vi "Magnetometer_Test_ReportGenerator.vi"() -> ()   [LabVIEW 2019]
uses:
  <vilib>/Utility/file.llb/Write Delimited Spreadsheet (string).vi
panel:
  in  "stop":bool
  out "error out":errorcluster
  out "Time 2":string
  out "X-Axis 2":string
  out "Time":string
  out "X-Axis":string
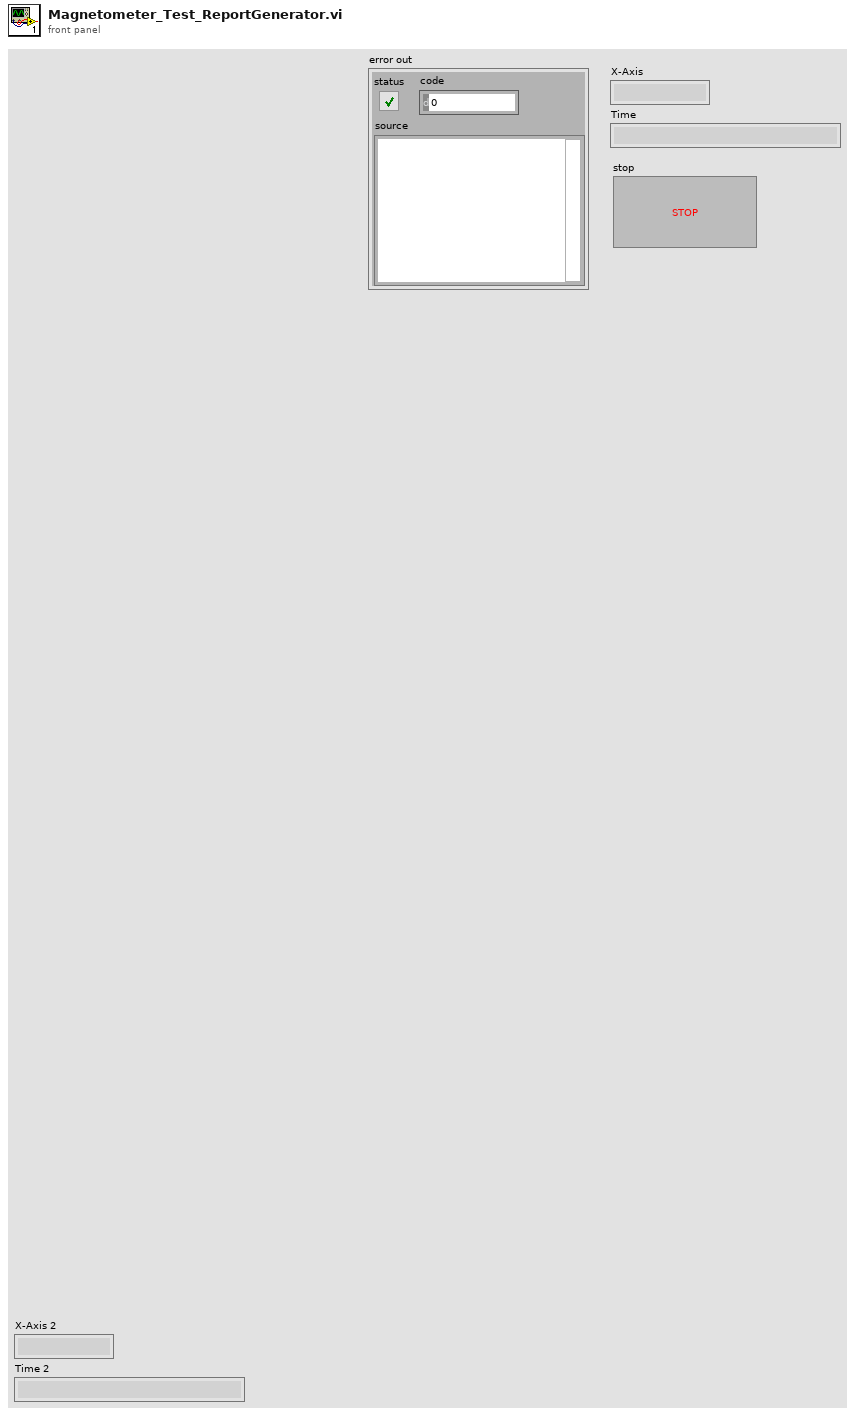
[diagram p1: front panel]
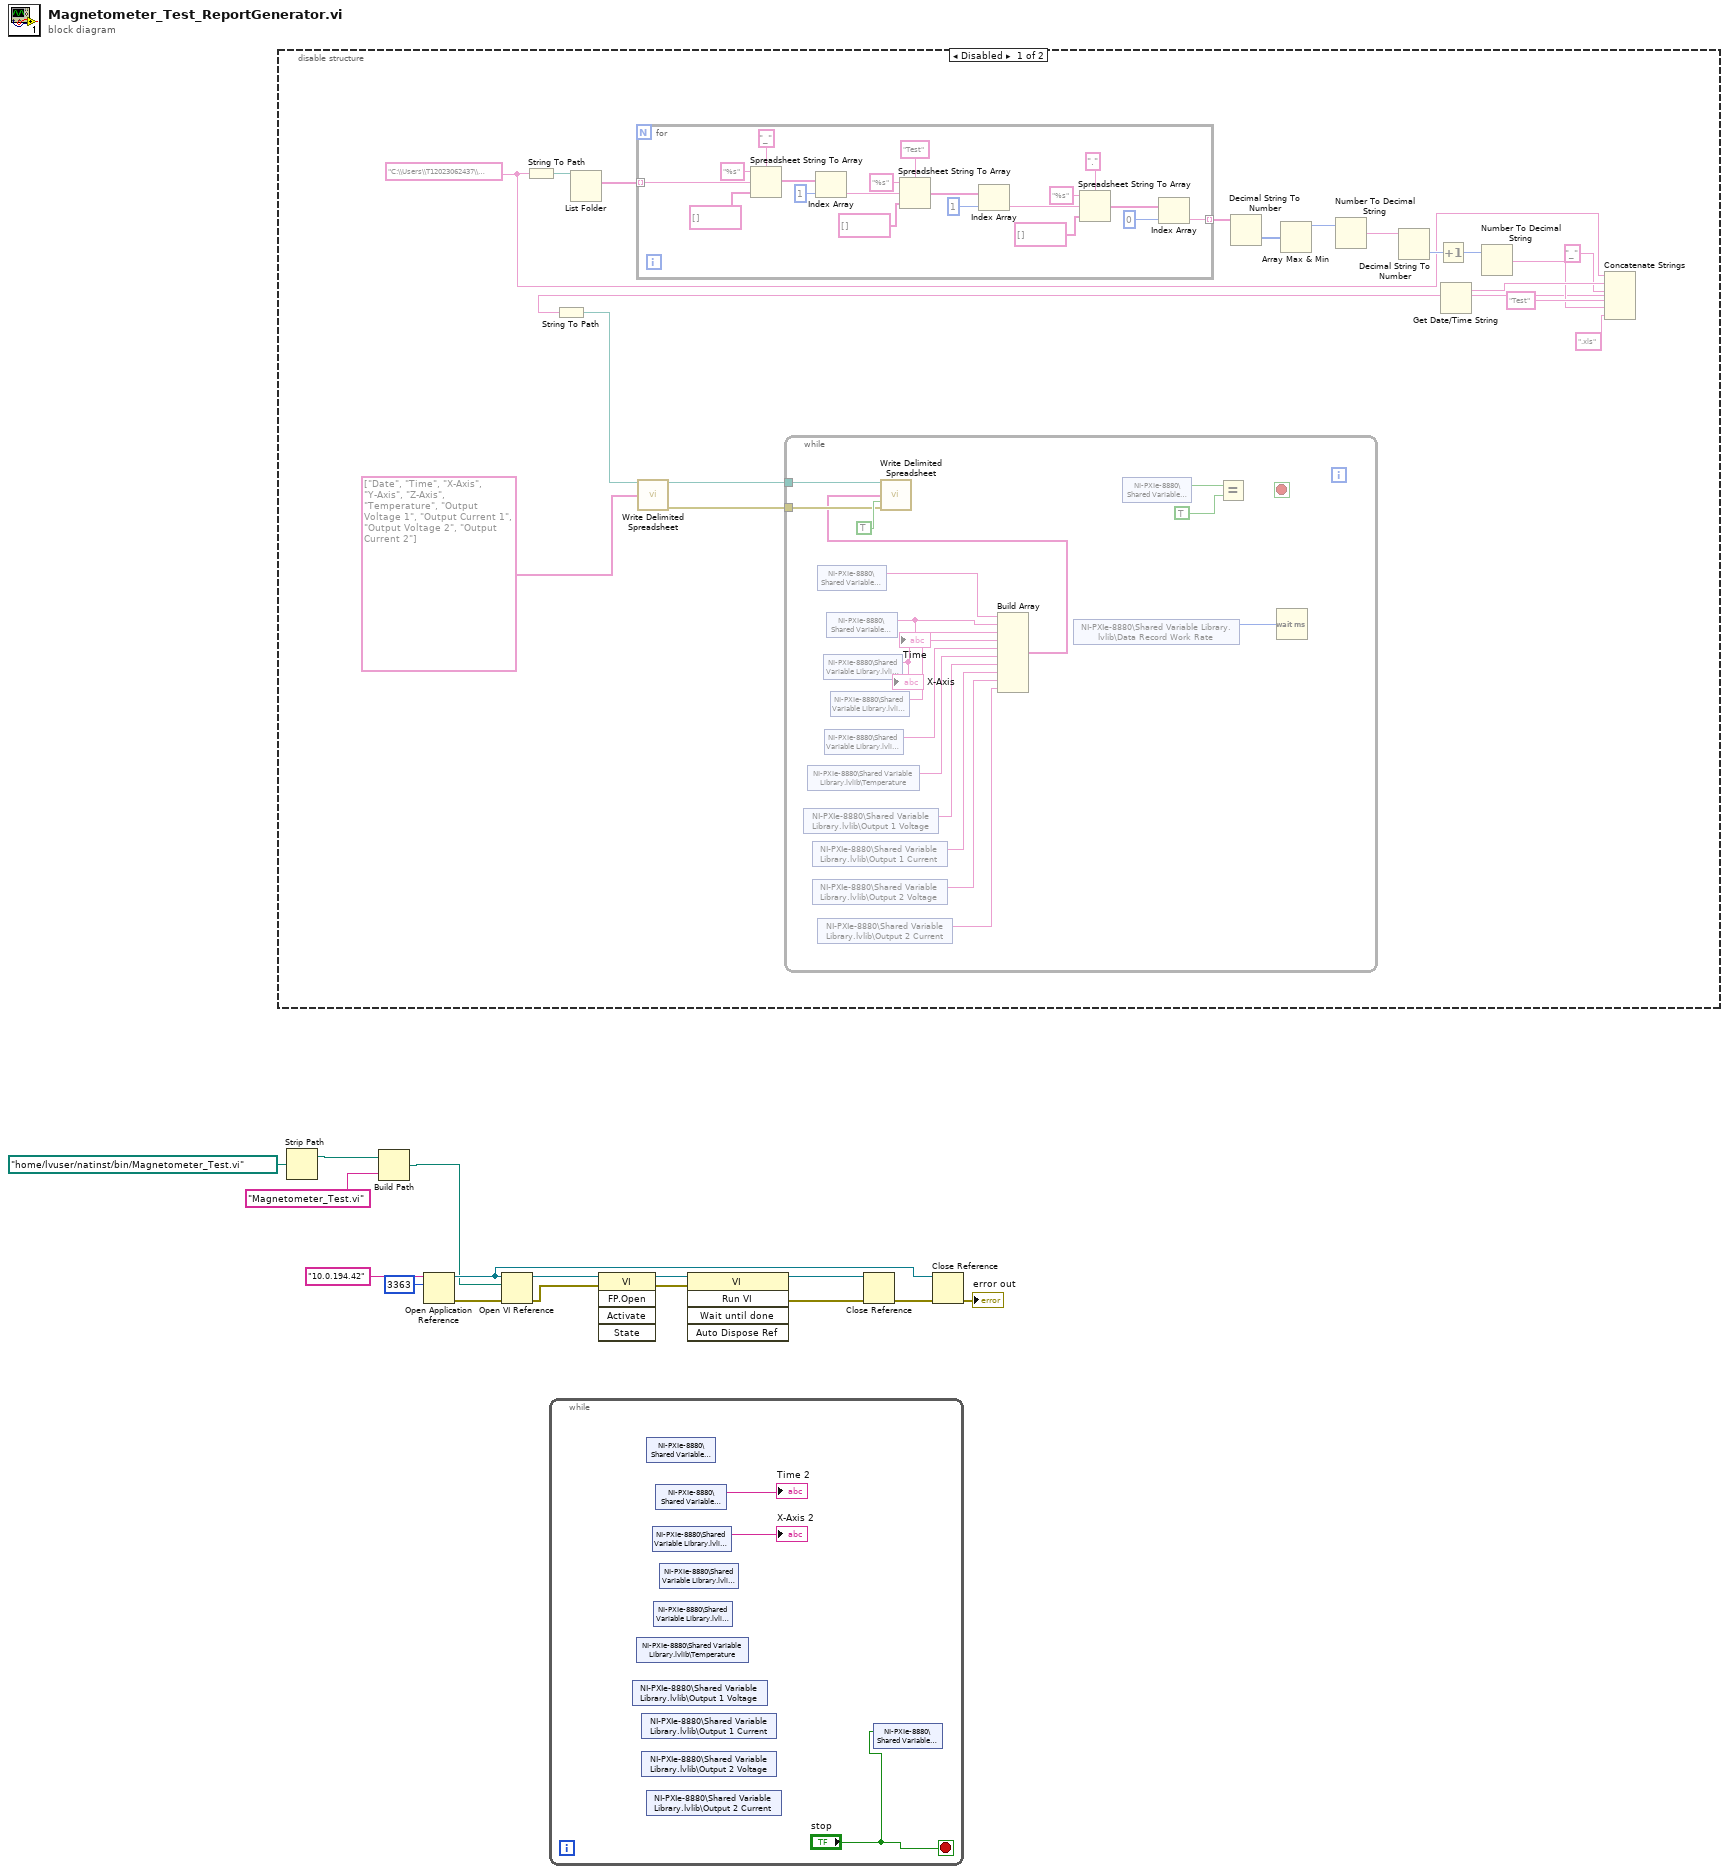
[diagram p0: block diagram]
diagram:
  n1 = disable-structure shown="Disabled" {
    frame Disabled {
      w19 = "C:\\Users\\T12023062437\\Desktop\\GKY Labview Models\\GKY Magnetometer Test Model Workspace\\Test Report\\"
      n2 = String To Path(string=w19) -> (path=w21:path)
      n3 = List Folder(path=w21) -> (filenames=w25:string[])  [unwired: 3 in, 3 out]
      n4 = for {
        tunnel: w25 -> [w39] mode=indexing
        tunnel: [w38] -> w24 mode=indexing
        n5 = Spreadsheet String To Array(delimiter (Tab)="_", format string="%s", spreadsheet string=w39, array type (2D Dbl)=string[] []) -> (array=w51:string[])
        n6 = Index Array(array=w51, index=1) -> (element=w52:string)
        n7 = Spreadsheet String To Array(delimiter (Tab)="Test", format string="%s", spreadsheet string=w52, array type (2D Dbl)=string[] []) -> (array=w36:string[])
        n8 = Index Array(array=w36, index=1) -> (element=w54:string)
        n9 = Spreadsheet String To Array(delimiter (Tab)=".", format string="%s", spreadsheet string=w54, array type (2D Dbl)=string[] []) -> (array=w53:string[])
        n10 = Index Array(array=w53, index=0) -> (element=w38:string)
      }
      n11 = Decimal String To Number(string=w24) -> (number=w23:i32[])  [unwired: 2 in, 1 out]
      n12 = Array Max & Min(array=w23) -> (max value=w22:i32)  [unwired: 3 out]
      n13 = Number To Decimal String(number=w22) -> (decimal integer string=w20:string)  [unwired: 1 in]
      n14 = Decimal String To Number(string=w20) -> (number=w30:i32)  [unwired: 2 in, 1 out]
      n15 = Increment(x=w30) -> (x+1=w29:i32)
      n16 = Get Date/Time String() -> (date string=w33:string)  [unwired: 3 in, 1 out]
      n17 = Number To Decimal String(number=w29) -> (decimal integer string=w28:string)  [unwired: 1 in]
      n18 = Concatenate Strings(w19, w33, "_" ("string"), "Test" ("string"), w28, ".xls" ("string")) -> (w27:string)
      n19 = String To Path(string=w27) -> (path=w17:path)
      n20 = call-poly <vilib>:"Write Delimited Spreadsheet.vi"("file path (dialog if empty)"=w17, "1D data"=string[] ["Date", "Time", "X-Axis", "Y-Axis", "Z-Axis", "Temperature", "Output Voltage 1", "Output Current 1", "Output Voltage 2", "Output Current 2"]) -> ("new file path (Not A Path if cancelled)"=w35:path, "error out"=w34:errorcluster)  [unwired: 12 in]
      n21 = while {
        tunnel: w35 -> [w73]
        tunnel: w34 -> [w71]
        stop <- w55 stop-if-true
        n22 = shared-variable "NI-PXIe-8880\\Shared Variable Library.lvlib\\Output 1 Voltage"() -> (w62:string)  [unwired: 1 in, 1 out]
        n23 = shared-variable "NI-PXIe-8880\\Shared Variable Library.lvlib\\Temperature"() -> (w63:string)  [unwired: 1 in, 1 out]
        n24 = shared-variable "NI-PXIe-8880\\Shared Variable Library.lvlib\\Output 1 Current"() -> (w61:string)  [unwired: 1 in, 1 out]
        n25 = shared-variable "NI-PXIe-8880\\Shared Variable Library.lvlib\\Output 2 Voltage"() -> (w60:string)  [unwired: 1 in, 1 out]
        n26 = shared-variable "NI-PXIe-8880\\Shared Variable Library.lvlib\\Date"() -> (w68:string)  [unwired: 1 in, 1 out]
        n27 = shared-variable "NI-PXIe-8880\\Shared Variable Library.lvlib\\Output 2 Current"() -> (w59:string)  [unwired: 1 in, 1 out]
        n28 = shared-variable "NI-PXIe-8880\\Shared Variable Library.lvlib\\X-Axis"() -> (w66:string)  [unwired: 1 in, 1 out]
        "X-Axis" <- w66
        n29 = shared-variable "NI-PXIe-8880\\Shared Variable Library.lvlib\\Z-Axis"() -> (w64:string)  [unwired: 1 in, 1 out]
        n30 = shared-variable "NI-PXIe-8880\\Shared Variable Library.lvlib\\Time"() -> (w67:string)  [unwired: 1 in, 1 out]
        "Time" <- w67
        n31 = shared-variable "NI-PXIe-8880\\Shared Variable Library.lvlib\\Y-Axis"() -> (w65:string)  [unwired: 1 in, 1 out]
        n32 = Build Array(w68, w67, w66, w65, w64, w63, w62, w61, w60, w59) -> (w58:string[])
        n33 = call-poly <vilib>:"Write Delimited Spreadsheet.vi"("file path (dialog if empty)"=w73, "1D data"=w58, "append to file? (new file:F)"=TRUE, "error in (no error)"=w71) -> ()  [unwired: 10 in, 2 out]
        n34 = shared-variable "NI-PXIe-8880\\Shared Variable Library.lvlib\\Data Record Work Rate"() -> (w57:u16)  [unwired: 1 in, 1 out]
        n35 = shared-variable "NI-PXIe-8880\\Shared Variable Library.lvlib\\Stop"() -> (w70:bool)  [unwired: 1 in, 1 out]
        n36 = Equal?(x=w70, y=TRUE) -> (x = y?=w56:bool)
        n37 = Wait (ms)(milliseconds to wait=w57) -> ()  [unwired: 1 out]
      }
    }
    frame Enabled {
    }
  }
  n38 = Strip Path(path=path "/home/lvuser/natinst/bin/Magnetometer_Test.vi") -> (stripped path=w5:path)  [unwired: 1 out]
  n39 = Build Path(base path=w5, name or relative path="Magnetometer_Test.vi") -> (appended path=w2:path)
  n40 = Open Application Reference(10:u16 3363 ("port number or service name (3363)"), 11:"10.0.194.42" ("machine name (\"\":  open local reference)")) -> (0:w13:errorcluster, 3:w7:refnum<vi>)  [unwired: 2 in]
  n41 = Open VI Reference(application reference (local)=w7, vi path=w2, error in (no error)=w13) -> (vi reference=w16:refnum<vi>, error out=w12:errorcluster)  [unwired: 3 in]
  n42 = while {
    stop <- "stop" stop-if-true
    n43 = shared-variable "NI-PXIe-8880\\Shared Variable Library.lvlib\\Output 1 Voltage"() -> ()  [unwired: 1 in, 2 out]
    n44 = shared-variable "NI-PXIe-8880\\Shared Variable Library.lvlib\\Temperature"() -> ()  [unwired: 1 in, 2 out]
    n45 = shared-variable "NI-PXIe-8880\\Shared Variable Library.lvlib\\Output 1 Current"() -> ()  [unwired: 1 in, 2 out]
    n46 = shared-variable "NI-PXIe-8880\\Shared Variable Library.lvlib\\Output 2 Voltage"() -> ()  [unwired: 1 in, 2 out]
    n47 = shared-variable "NI-PXIe-8880\\Shared Variable Library.lvlib\\Date"() -> ()  [unwired: 1 in, 2 out]
    n48 = shared-variable "NI-PXIe-8880\\Shared Variable Library.lvlib\\Output 2 Current"() -> ()  [unwired: 1 in, 2 out]
    n49 = shared-variable "NI-PXIe-8880\\Shared Variable Library.lvlib\\X-Axis"() -> (→"X-Axis 2":string)  [unwired: 1 in, 1 out]
    n50 = shared-variable "NI-PXIe-8880\\Shared Variable Library.lvlib\\Z-Axis"() -> ()  [unwired: 1 in, 2 out]
    n51 = shared-variable "NI-PXIe-8880\\Shared Variable Library.lvlib\\Time"() -> (→"Time 2":string)  [unwired: 1 in, 1 out]
    n52 = shared-variable "NI-PXIe-8880\\Shared Variable Library.lvlib\\Y-Axis"() -> ()  [unwired: 1 in, 2 out]
    n53 = shared-variable "NI-PXIe-8880\\Shared Variable Library.lvlib\\Stop"("stop") -> ()  [unwired: 1 in, 1 out]
  }
  n54 = invoke class="VI" method="FP.Open"(reference=w16, error in=w12) -> (reference out=w15:refnum<vi>, error out=w11:errorcluster)  [unwired: 3 in, 3 out]
  n55 = invoke class="VI" method="Run VI"(reference=w15, error in=w11) -> (reference out=w14:refnum<vi>, error out=w10:errorcluster)  [unwired: 3 in, 3 out]
  n56 = Close Reference(reference=w14, error in (no error)=w10) -> (error out=w8:errorcluster)
  n57 = Close Reference(reference=w7, error in (no error)=w8) -> (error out=→"error out":errorcluster)
